vi "Plugin - Sine Graph.vi"() -> ()   [LabVIEW 2023]
doc: "Subpanel Plugin VI that displays a sine wave with varying phase on a waveform graph."
panel:
  out "Waveform Graph":dynamicdata(graph)
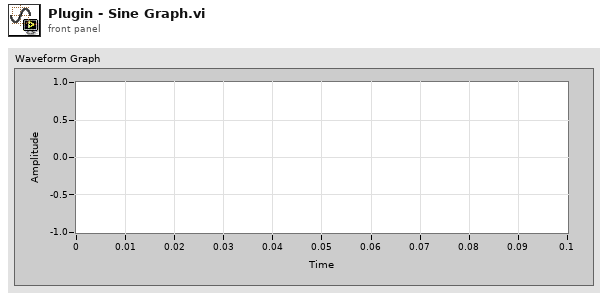
[diagram p1: front panel]
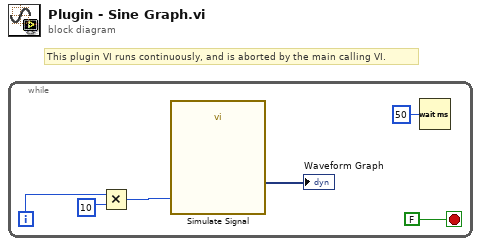
[diagram p0: block diagram]
diagram:
  # "This plugin VI runs continuously, and is aborted by the main calling VI."
  n1 = while {
    i -> [w5]
    stop <- FALSE stop-if-true
    n2 = Multiply(x=w5, y=10) -> (x*y=w1:i32)
    n3 = call "Simulate Signal"("Phase"=w1) -> ("Sine"=→"Waveform Graph":dynamicdata)  [unwired: 13 in, 1 out]
    n4 = Wait (ms)(milliseconds to wait=u32 50) -> ()  [unwired: 1 out]
  }
